vi "Find Most Recently Modified File.vi"(7 "error in (no error)":errorcluster, 9 "Pattern":string, 10 "Directory":path) -> (0 "error out":errorcluster, 2 "2nd Most Recent File Path":path, 3 "Most Recent File Path":path)   [LabVIEW 2013]
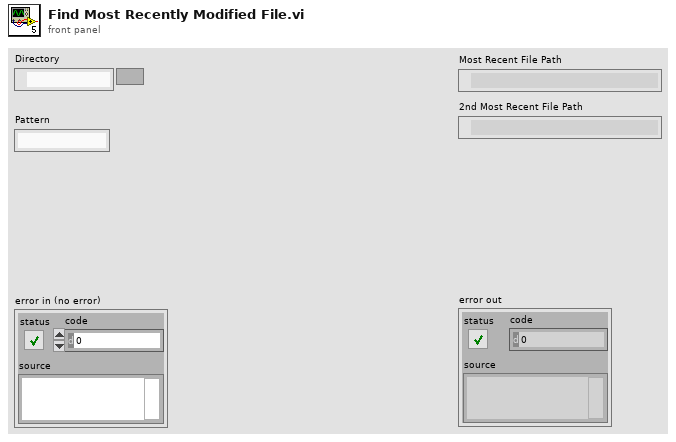
[diagram p1: front panel]
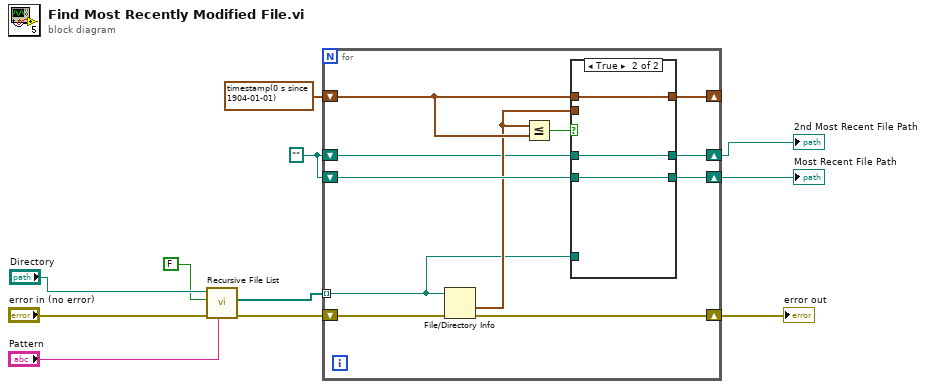
[diagram p0: block diagram]
diagram:
  w8 = path ""
  n1 = call <vilib>:"Recursive File List.vi"("pattern"="Pattern", "error in (no error)"="error in (no error)", "Treat LLBs as Folders?"=FALSE, "Folder Path"="Directory") -> ("error out"=w2:errorcluster, "All Files in Dir"=w1:path[])  [unwired: 3 in, 3 out]
  n2 = for {
    shift-right: [w21] -> w10
    shift-left: w2 -> [w22]
    shift-right: [w16] -> w9
    shift-left: w8 -> [w18]
    shift-right: [w19] -> _
    shift-left: timestamp(0 s since 1904-01-01) ("last mod") -> [w20]
    shift-right: [w13] -> w7
    shift-left: w8 -> [w14]
    tunnel: w1 -> [w12] mode=indexing
    n3 = File/Directory Info(path=w12, error in=w22) -> (last mod=w15:timestamp, error out=w21:errorcluster)  [unwired: 5 out]
    n4 = Less Or Equal?(x=w15, y=w20) -> (x <= y?=w17:bool)
    n5 = case shown="True" w17 {
      tunnel: w20 -> [_ w28]
      tunnel: [w24 w28] -> w19
      tunnel: w18 -> [w23 w27]
      tunnel: [w25 w27] -> w16
      tunnel: w12 -> [w25 _]
      tunnel: w15 -> [w24 _]
      tunnel: w14 -> [_ w26]
      tunnel: [w23 w26] -> w13
      frame False {
      }
      frame True {
      }
    }
  }
  "error out" <- w10
  "Most Recent File Path" <- w9
  "2nd Most Recent File Path" <- w7
